vi "DriverStation Set Display.vi"(8 "error in (no error)":errorcluster, 10 "display string":string, 11 "reset":bool) -> (0 "error out":errorcluster)   [LabVIEW 2026, in "MrcLib.lvlib"]
doc: "If Reset it true, it first resets the replay state of the Driver Station.\nIt then updates the Driver Station to display the text message."
uses:
  MrcLib.lvlib
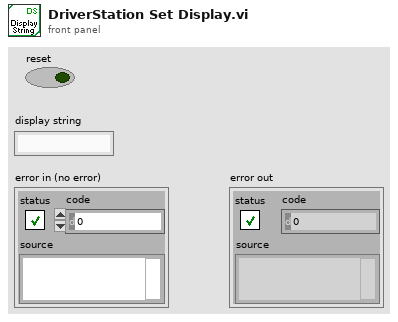
[diagram p1: front panel]
types:
  T1 = typedef "MRC String.ctl" = cluster{"pointer":u64, "length":u64}
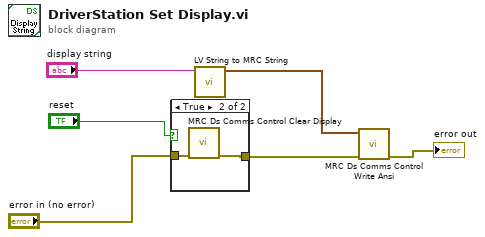
[diagram p0: block diagram]
diagram:
  n1 = case shown="True" "reset" {
    tunnel: "error in (no error)" -> [w7 w9]
    tunnel: [w7 w8] -> w5
    frame False {
    }
    frame True {
      n2 = call "MRC Ds Comms Control Clear Display.vi"("error in (no error)"=w9) -> ("error out"=w8:errorcluster)  [unwired: 10 in]
    }
  }
  n3 = call "LV String to MRC String.vi"("LV String"="display string") -> ("MRC String"=w1:T1)  [unwired: 10 in]
  n4 = call "MRC Ds Comms Control Write Ansi.vi"("error in (no error)"=w5, "text"=w1) -> ("error out"=→"error out":errorcluster)  [unwired: 9 in]
